vi "red buoy2.0.vi"(6 "error in (no error)":errorcluster, 7 "Cluster":cluster{"Min Radius":sgl, "Max Radius":sgl}={"Min Radius"=7.0, "Max Radius"=50.0}, 9 "Image":T2) -> (0 "error out":errorcluster, 1 "Circles Data (calibrated)":T1(array[cluster]), 2 "Nb Circles":i32, 3 "Image Out":T2(plugin-control))   [LabVIEW 2009]
uses:
  <vilib>/vision/Image Controls.llb/IMAQ Image.ctl
  <vilib>/vision/NI_Vision_Development_Module.lvlib
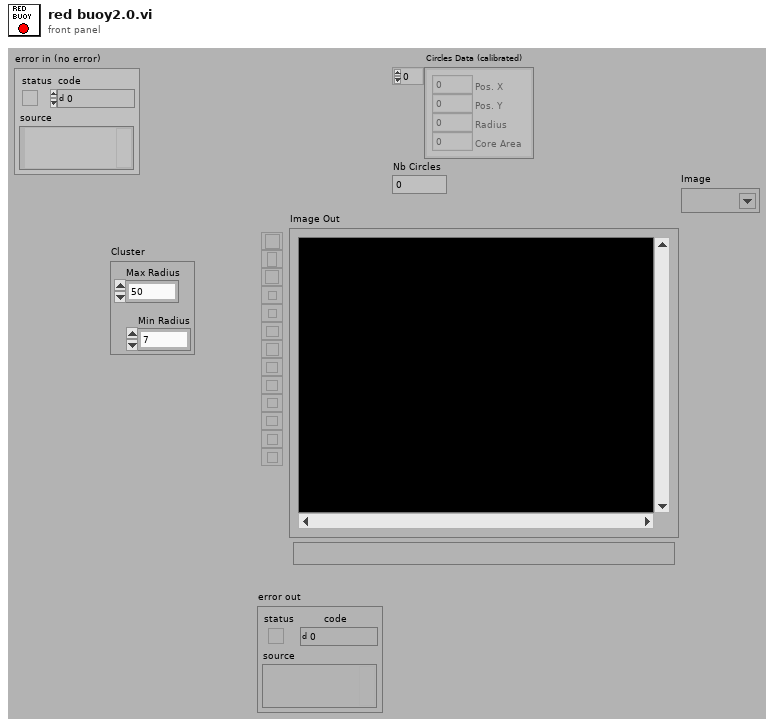
[diagram p1: front panel]
types:
  T1 = cluster{"Pos. X":i32, "Pos. Y":i32, "Radius":i32, "Core Area":i32}[]
  T2 = typedef "IMAQ Image.ctl" = refnum<image>
  T3 = enum32{"AutoM", "Close", "Dilate", "Erode", "Gradient", "Gradient out", "Gradient in", "Hit miss", "Open", "PClose", "POpen", "Thick", "Thin"}
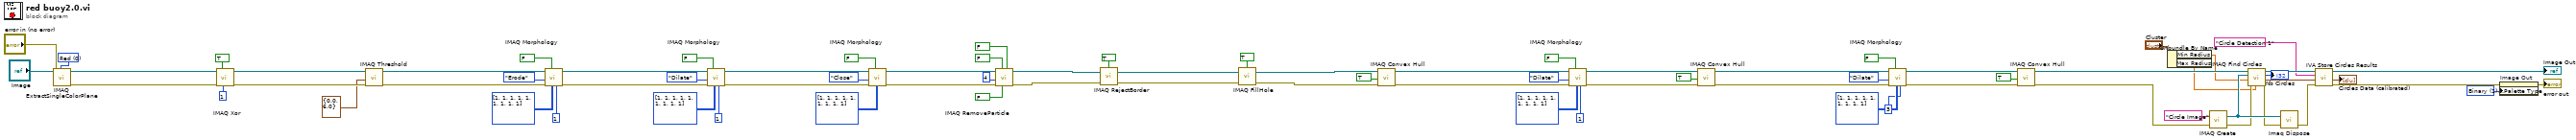
[diagram p0: block diagram]
diagram:
  w9 = u32 1 items=["Grayscale", "Binary", "Gradient", "Rainbow", "Temperature", "User Defined"] ("Palette")
  w78 = 0 items=["Red", "Green", "Blue", "Hue", "Saturation", "Luminance", "Value", "Intensity"] ("Color Plane")
  n1 = call "IMAQ ExtractSingleColorPlane"("Color Plane"=w78, "error in (no error)"="error in (no error)", "Image Src"="Image") -> ("error out"=w77:errorcluster, "Image Dst Out"=w74:T2)  [unwired: 1 in, 6 out]
  n2 = call "IMAQ Xor"("Constant"=1, "Xor/Xnor (Xor)"=TRUE, "error in (no error)"=w77, "Image Src A"=w74) -> ("error out"=w73:errorcluster, "Image Dst Out"=w71:T2)  [unwired: 2 in, 4 out]
  n3 = call "IMAQ Threshold"("error in (no error)"=w73, "Range"=cluster{"Lower value":sgl, "Upper value":sgl} {"Lower value"=0.0, "Upper value"=6.0}, "Image Src"=w71) -> ("error out"=w70:errorcluster, "Image Dst Out"=w65:T2)  [unwired: 3 in, 4 out]
  n4 = call "IMAQ Morphology"("Number of iterations (1)"=1, "Structuring Element"=i32[][] [[1, 1, 1], [1, 1, 1], [1, 1, 1]], "Square/Hexa (Square)"=FALSE, "error in (no error)"=w70, "Operation"=T3."Erode", "Image Src"=w65) -> ("error out"=w64:errorcluster, "Image Dst Out"=w59:T2)  [unwired: 1 in, 3 out]
  n5 = call "IMAQ Morphology"("Number of iterations (1)"=1, "Structuring Element"=i32[][] [[1, 1, 1], [1, 1, 1], [1, 1, 1]], "Square/Hexa (Square)"=FALSE, "error in (no error)"=w64, "Operation"=T3."Dilate", "Image Src"=w59) -> ("error out"=w58:errorcluster, "Image Dst Out"=w54:T2)  [unwired: 1 in, 3 out]
  n6 = call "IMAQ Morphology"("Structuring Element"=i32[][] [[1, 1, 1], [1, 1, 1], [1, 1, 1]], "Square/Hexa (Square)"=FALSE, "error in (no error)"=w58, "Operation"=T3."Close", "Image Src"=w54) -> ("error out"=w53:errorcluster, "Image Dst Out"=w48:T2)  [unwired: 2 in, 3 out]
  n7 = call "IMAQ RemoveParticle"("Connectivity 4/8 (8)"=FALSE, "Low Pass/High Pass (Low)"=FALSE, "Square/Hexa (Square)"=FALSE, "error in (no error)"=w53, "Number of Erosion"=4, "Image Src"=w48) -> ("error out"=w47:errorcluster, "Image Dst Out"=w45:T2)  [unwired: 1 in, 3 out]
  n8 = call "IMAQ RejectBorder"("error in (no error)"=w47, "Image Src"=w45, "Connectivity 4/8 (8)"=TRUE) -> ("error out"=w44:errorcluster, "Image Dst Out"=w42:T2)  [unwired: 1 in, 2 out]
  n9 = call "IMAQ FillHole"("error in (no error)"=w44, "Image Src"=w42, "Connectivity 4/8 (8)"=TRUE) -> ("error out"=w41:errorcluster, "Image Dst Out"=w40:T2)  [unwired: 1 in, 2 out]
  n10 = call "IMAQ Convex Hull"("error in (no error)"=w41, "Connectivity 4/8 (8)"=TRUE, "Image Src"=w40) -> ("error out"=w38:errorcluster, "Image Dst Out"=w33:T2)  [unwired: 1 in, 6 out]
  n11 = call "IMAQ Morphology"("Number of iterations (1)"=1, "Structuring Element"=i32[][] [[1, 1, 1], [1, 1, 1], [1, 1, 1]], "Square/Hexa (Square)"=FALSE, "error in (no error)"=w38, "Operation"=T3."Dilate", "Image Src"=w33) -> ("error out"=w32:errorcluster, "Image Dst Out"=w31:T2)  [unwired: 1 in, 3 out]
  n12 = call "IMAQ Convex Hull"("error in (no error)"=w32, "Connectivity 4/8 (8)"=TRUE, "Image Src"=w31) -> ("error out"=w29:errorcluster, "Image Dst Out"=w24:T2)  [unwired: 1 in, 6 out]
  n13 = call "IMAQ Morphology"("Number of iterations (1)"=3, "Structuring Element"=i32[][] [[1, 1, 1], [1, 1, 1], [1, 1, 1]], "Square/Hexa (Square)"=FALSE, "error in (no error)"=w29, "Operation"=T3."Dilate", "Image Src"=w24) -> ("error out"=w23:errorcluster, "Image Dst Out"=w22:T2)  [unwired: 1 in, 3 out]
  n14 = call "IMAQ Convex Hull"("error in (no error)"=w23, "Connectivity 4/8 (8)"=TRUE, "Image Src"=w22) -> ("error out"=w20:errorcluster, "Image Dst Out"=w13:T2)  [unwired: 1 in, 6 out]
  n15 = Unbundle By Name("Cluster") -> ("Min Radius"=w2:sgl, "Max Radius"=w1:sgl)
  n16 = call "IMAQ Create"("Image Name"="Circle Image", "error in (no error)"=w20) -> ("New Image"=w18:T2, "error out"=w17:errorcluster)  [unwired: 2 in, 1 out]
  n17 = call "IMAQ Find Circles"("Max Radius"=w1, "error in (no error)"=w17, "Min Radius"=w2, "Image Dst"=w18, "Image Src"=w13) -> ("error out"=w16:errorcluster, "Circles Data"=w11:T1, "Nb Circles"=→"Nb Circles":i32)  [unwired: 4 out]
  n18 = call "Imaq Dispose"("Image"=w18, "error in (no error)"=w16) -> ("error out"=w15:errorcluster)  [unwired: 1 in, 3 out]
  n19 = call <vilib>:"IVA Store Circles Results.vi"("error in (no error)"=w15, "Circles Data"=w11, "Step Name"="Circle Detection 1", "Image in"=w13) -> ("error out"=w14:errorcluster, "Circles Data (calibrated)"=→"Circles Data (calibrated)":T1, "Image dup"=→"Image Out":T2)  [unwired: 5 out]
  n20 = property on="Image Out" class="ImageControl"(error in=w14, "Palette:Palette Type"=w9) -> (error out=→"error out":errorcluster)  [unwired: 1 in, 1 out]
